vi "MatlabExperiment.vi"() -> ()   [LabVIEW 2017]
uses:
  C:/Code/CMCryoSysCode/CSharp/MatlabEditor/MatlabEditor/bin/Debug/MatlabEditor.dll
  CMCryoSysCode/CSharp/MatlabEditor/MatlabEditor/bin/Debug/MatlabEditor.dll
panel:
  in  "ScriptFile":path=path "experiment.m"
  out "information_text":string="Run function file to be used when executing the data. Function file should have three functions (init, loop, complete). The function file CANNOT have a function with the same name of the file."
  in  "MEditor":refnum<k24>(container)
  out "Error Info":string
  out "ExperimentEventReg":refnum<event-registration>
  out "ExperimentEvents":refnum<user-event>
  in  "btnShowCode":bool
  out "CodeSplitterLastPosition":i32
  in  "btnUpdateProperties":bool
  in  "btnCompile":bool
  in  "btnRUN":bool
  in  "SomeStringProp":string
  in  "SomeArrayProp":dbl[](array[numeric])
  in  "SomeProperty":dbl
  out "ExperimentID":string
  out "hasCompileErrors":bool
  out "IsBusy":bool
  out "IsRunning":bool
  # "Experiment ID"
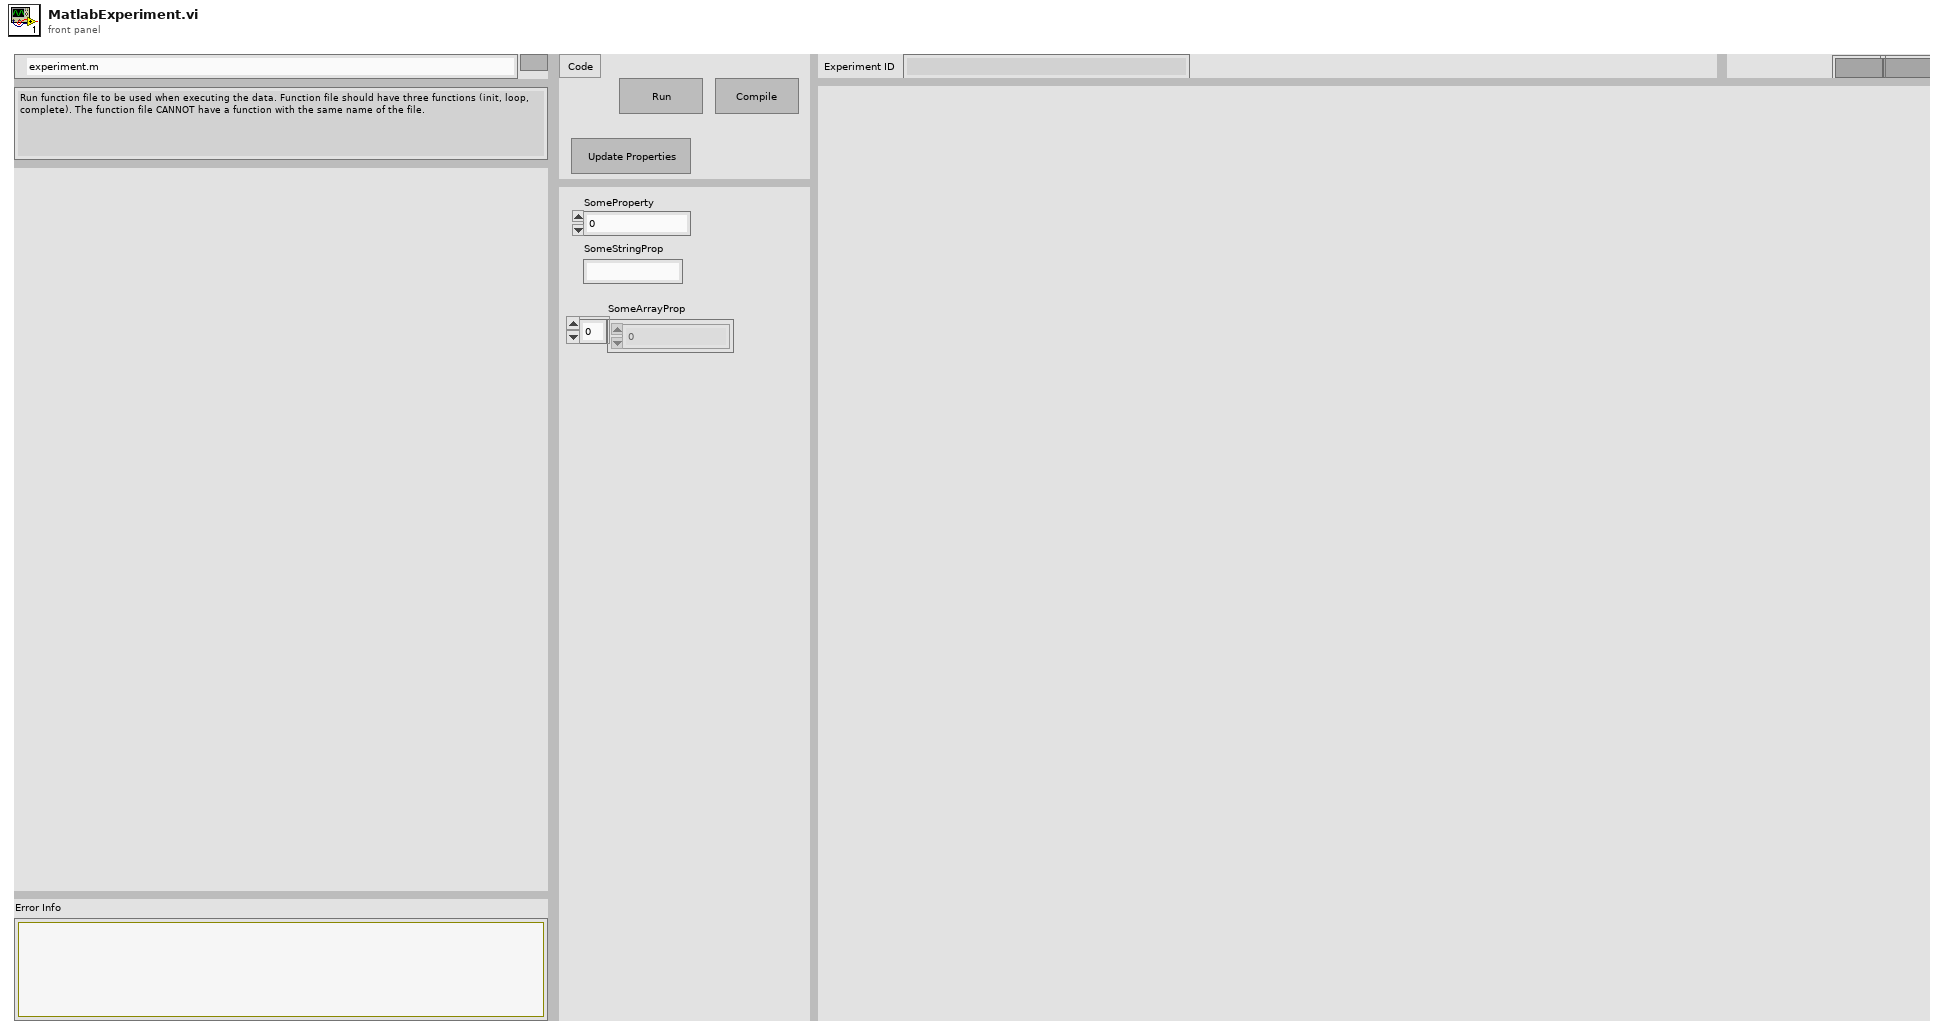
[diagram p1: front panel]
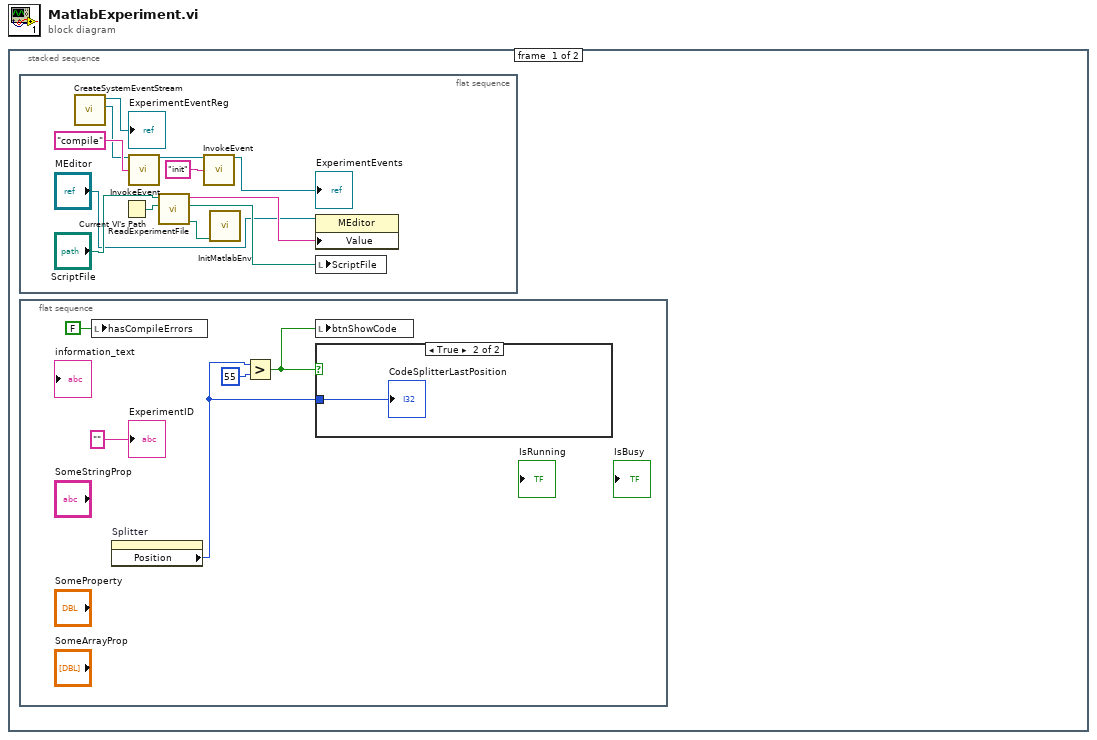
[diagram p0: block diagram]
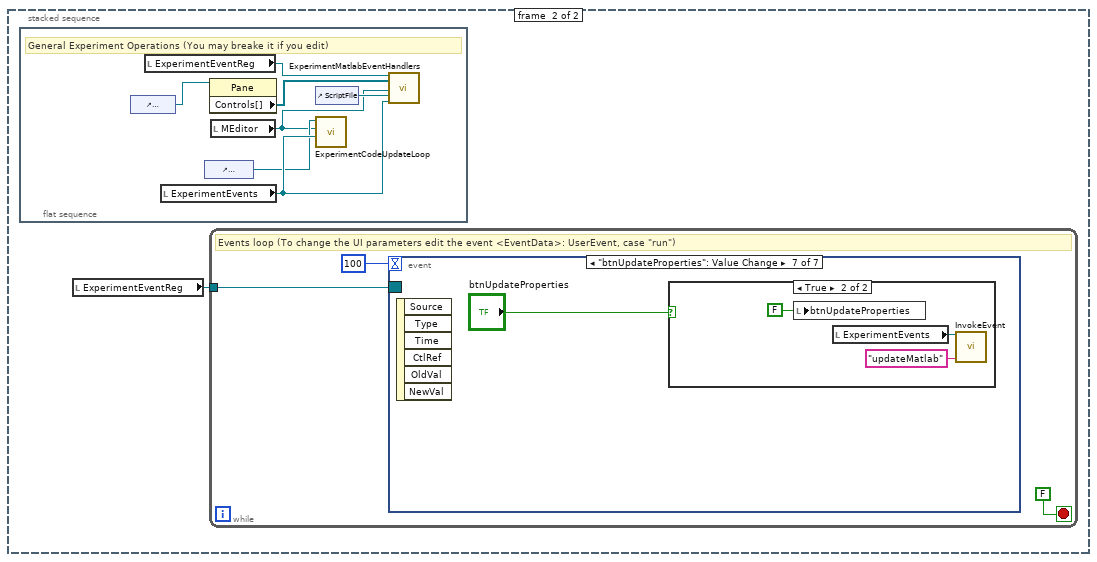
[diagram p3: hidden frame]
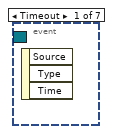
[diagram p4: hidden frame]
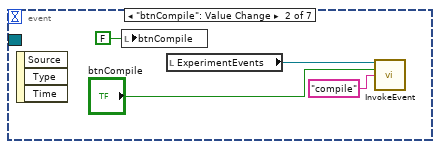
[diagram p5: hidden frame]
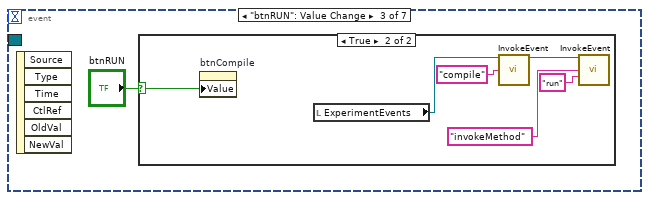
[diagram p6: hidden frame]
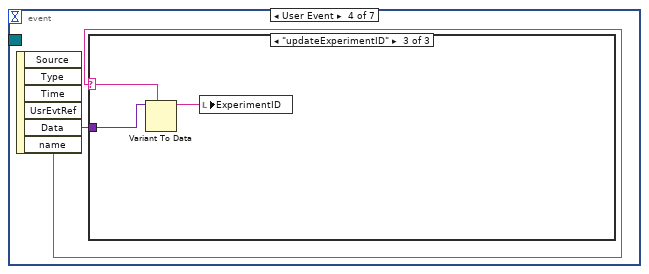
[diagram p8: hidden frame]
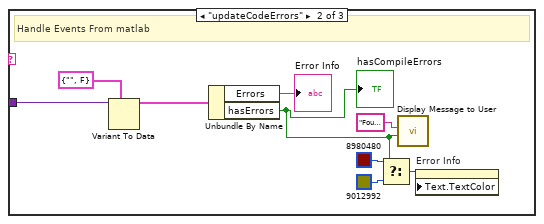
[diagram p10: hidden frame]
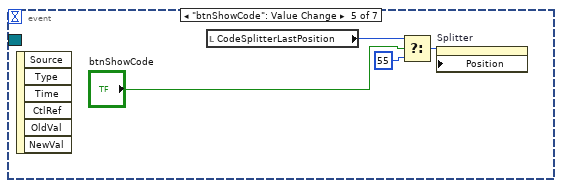
[diagram p11: hidden frame]
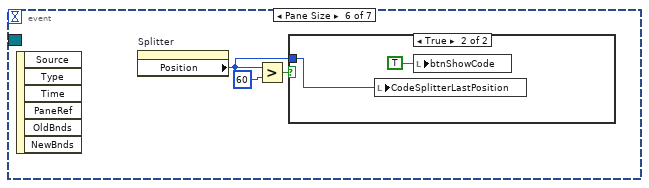
[diagram p12: hidden frame]
diagram:
  n1 = stacked-sequence {
    frame #0 {
      n2 = flat-sequence {
        frame #0 {
          n3 = call "CreateSystemEventStream.vi"() -> ("ExperimentEvents"=w3:refnum<user-event>, "Event Registration Refnum out"=→"ExperimentEventReg":refnum<event-registration>)  [unwired: 10 in]
          n4 = Current VI's Path() -> (path=w10:path)
          n5 = call "InvokeEvent.vi"("User Event in"=w3, "name"="compile") -> ("user event out"=w2:refnum<user-event>)  [unwired: 12 in, 1 out]
          n6 = call "ReadExperimentFile.vi"("BaseSearchPath"=w10, "ScriptFile"="ScriptFile") -> ("Working Directory"=w7:path, "FilePath"=w9:path, "String"=w12:string)  [unwired: 7 in]
          n7 = call "InvokeEvent.vi"("User Event in"=w2, "name"="init") -> ("user event out"=→"ExperimentEvents":refnum<user-event>)  [unwired: 12 in, 1 out]
          n8 = call "InitMatlabEnv.vi"("Matlab Working Directory"=w7) -> ()  [unwired: 11 in]
          n9 = property class="MEditor"(reference="MEditor", "Value"=w12) -> ()  [unwired: 1 in, 2 out]
          n10 = local write "ScriptFile"(w9) -> ()
        }
      }
      n11 = flat-sequence {
        frame #0 {
          n12 = local write "hasCompileErrors"(FALSE ("hasCompileErrors")) -> ()
          n13 = property on="Splitter" class="Splitter"() -> ("Position"=w15:i32)  [unwired: 2 in, 2 out]
          n14 = Greater?(x=w15, y=55) -> (0:w13:bool)
          n15 = local write "btnShowCode"(w13) -> ()
          n16 = case shown="True" w13 {
            tunnel: w15 -> [_ w18]
            frame False {
            }
            frame True {
              "CodeSplitterLastPosition" <- w18
            }
          }
          "ExperimentID" <- "" ("ExperimentID")
        }
      }
    }
    frame #1 {
      n17 = flat-sequence {
        frame #0 {
          # "General Experiment Operations (You may breake it if you edit)"
          n18 = control-ref of="ControlsPane"() -> (w22:refnum<vi>)
          n19 = local read "ExperimentEventReg"() -> (w25:refnum<event-registration>)
          n20 = local read "ExperimentEvents"() -> (w26:refnum<user-event>)
          n21 = control-ref of="ExperimentID"() -> (w24:refnum<vi>)
          n22 = property class="Pane"(reference=w22) -> ("Controls[]"=w21:refnum<vi>[])  [unwired: 1 in, 2 out]
          n23 = local read "MEditor"() -> (w20:refnum<k24>)
          n24 = control-ref of="ScriptFile"() -> (w23:refnum<vi>)
          n25 = call "ExperimentCodeUpdateLoop.vi"("EventData in"=w26, "MEditor"=w20, "ExperimentID"=w24) -> ()  [unwired: 9 in]
          n26 = call "ExperimentMatlabEventHandlers.vi"("Event Registration Refnum in"=w25, "Controls[]"=w21, "MEditor"=w20, "ScriptFile"=w23, "user event in"=w26) -> ()  [unwired: 15 in]
        }
      }
      n27 = local read "ExperimentEventReg"() -> (w19:refnum<event-registration>)
      n28 = while {
        tunnel: w19 -> [w27]
        stop <- FALSE stop-if-true
        # "Events loop (To change the UI parameters edit the event <EventData>: UserEvent, case \"run\")"
        n29 = event shown="[6] \"btnUpdateProperties\": Value Change" {
          selector: w27 -> [_ _ _ _ _ _ _]
          dyn-events: _ -> [_ _ _ _ _ _ _]
          timeout: 100 -> [_ _ _ _ _ _ _]
          event Timeout {
            n30 = event-data() -> ()  [unwired: 1 in, 3 out]
          }
          event "btnCompile": Value Change {
            n31 = event-data() -> ()  [unwired: 1 in, 3 out]
            n32 = local write "btnCompile"(FALSE ("btnCompile")) -> ()
            n33 = local read "ExperimentEvents"() -> (w30:refnum<user-event>)
            n34 = call "InvokeEvent.vi"("User Event in"=w30, "Invoke?"="btnCompile", "name"="compile") -> ()  [unwired: 11 in, 2 out]
          }
          event "btnRUN": Value Change {
            n35 = event-data() -> ()  [unwired: 1 in, 6 out]
            n36 = case shown="True" "btnRUN" {
              selector: "btnRUN" -> [_ w38]
              frame False {
              }
              frame True {
                n37 = property on="btnCompile" class="Bool (strict)"("Value"=w38) -> ()  [unwired: 2 in, 2 out]
                n38 = local read "ExperimentEvents"() -> (w35:refnum<user-event>)
                n39 = call "InvokeEvent.vi"("User Event in"=w35, "name"="compile") -> ("user event out"=w39:refnum<user-event>)  [unwired: 12 in, 1 out]
                n40 = call "InvokeEvent.vi"("User Event in"=w39, "name"="invokeMethod", "Data"="run" ("name")) -> ()  [unwired: 11 in, 2 out]
              }
            }
          }
          event User Event {
            n41 = event-data() -> ("Data"=w41:variant, "name"=w42:string)  [unwired: 1 in, 4 out]
            n42 = case shown="\"updateExperimentID\"" w42 {
              selector: w42 -> [_ _ w52]
              tunnel: w41 -> [_ w51 w54]
              frame "False", Default {
              }
              frame "updateCodeErrors" {
                # "Handle Events From matlab"
                n43 = Variant To Data(type=cluster{"Errors":string, "hasErrors":bool} {"Errors"="", "hasErrors"=FALSE}, Variant=w51) -> (data=w49:cluster{"Errors":string, "hasErrors":bool})  [unwired: 1 in, 1 out]
                n44 = Unbundle By Name(w49) -> ("Errors"=→"Error Info":string, "hasErrors"=w43:bool)
                "hasCompileErrors" <- w43
                n45 = Select(t=u32 8980480, s=w43, f=u32 9012992) -> (s? t:f=w47:u32)
                n46 = call "Display Message to User"("Enable"=w43, "Message"="Found errors in the code." ("string")) -> ()  [unwired: 8 in, 2 out]
                n47 = property on="Error Info" class="Str"("Text.TextColor"=w47) -> ()  [unwired: 2 in, 2 out]
              }
              frame "updateExperimentID" {
                n48 = Variant To Data(type=w52, Variant=w54) -> (data=w53:string)  [unwired: 1 in, 1 out]
                n49 = local write "ExperimentID"(w53) -> ()
              }
            }
          }
          event "btnShowCode": Value Change {
            n50 = event-data() -> ()  [unwired: 1 in, 6 out]
            n51 = local read "CodeSplitterLastPosition"() -> (w56:i32)
            n52 = Select(t=w56, s="btnShowCode", f=55) -> (s? t:f=w57:i32)
            n53 = property on="Splitter" class="Splitter"("Position"=w57) -> ()  [unwired: 2 in, 2 out]
          }
          event Pane Size {
            n54 = event-data() -> ()  [unwired: 1 in, 6 out]
            n55 = property on="Splitter" class="Splitter"() -> ("Position"=w61:i32)  [unwired: 2 in, 2 out]
            n56 = Greater?(x=w61, y=60) -> (0:w59:bool)
            n57 = case shown="True" w59 {
              tunnel: w61 -> [_ w62]
              frame False {
              }
              frame True {
                n58 = local write "CodeSplitterLastPosition"(w62) -> ()
                n59 = local write "btnShowCode"(TRUE ("btnShowCode")) -> ()
              }
            }
          }
          event "btnUpdateProperties": Value Change {
            n60 = event-data() -> ()  [unwired: 1 in, 6 out]
            n61 = case shown="True" "btnUpdateProperties" {
              frame False {
              }
              frame True {
                n62 = local write "btnUpdateProperties"(FALSE ("btnUpdateProperties")) -> ()
                n63 = local read "ExperimentEvents"() -> (w65:refnum<user-event>)
                n64 = call "InvokeEvent.vi"("User Event in"=w65, "name"="updateMatlab") -> ()  [unwired: 12 in, 2 out]
              }
            }
          }
        }
      }
    }
  }
